vi "PSVCH_Check Double Quotation Marks.vi"(8 "Error In (no error)":errorcluster, 11 "String":string) -> (0 "Error Out":errorcluster, 2 "\"Tag\"[]":string[](array[string]), 3 "Error?":bool)   [LabVIEW 2016]
uses:
  <vilib>/regexp/Match Regular Expression.xnode
panel:
  # "Data In"
  # "Data Out"
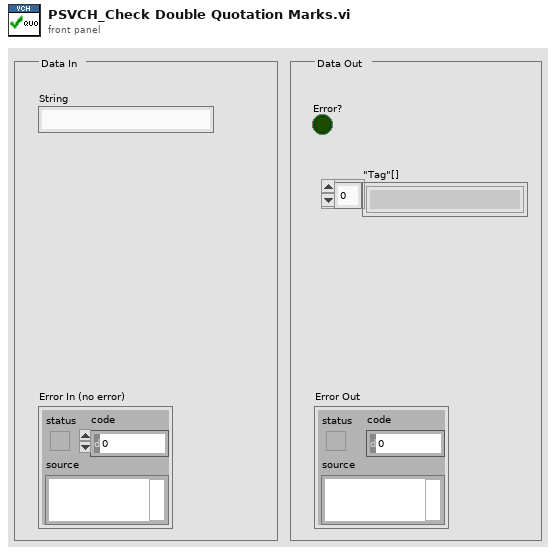
[diagram p1: front panel]
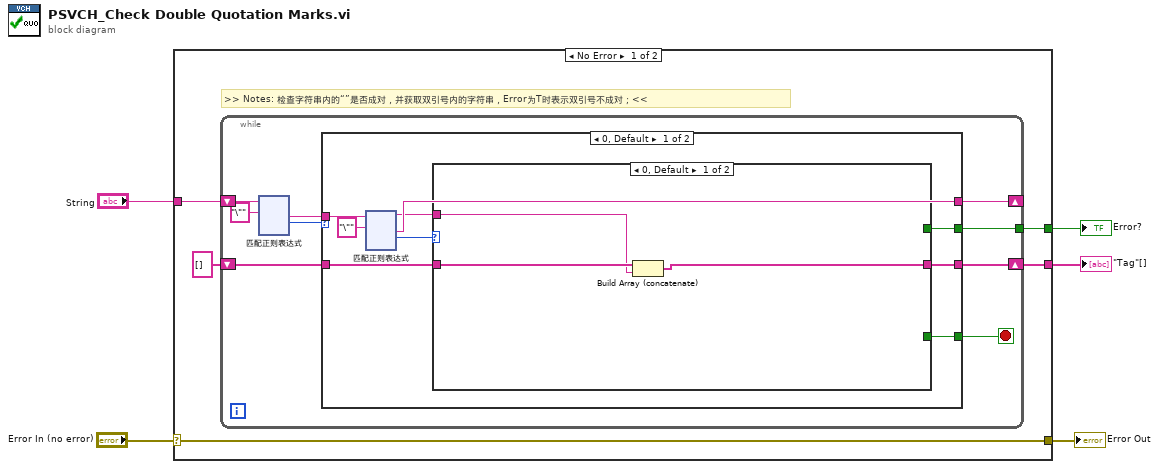
[diagram p0: block diagram]
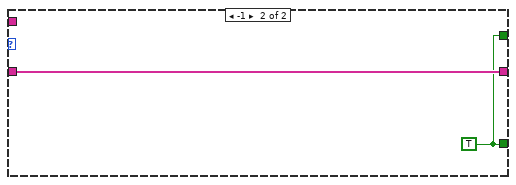
[diagram p2: hidden frame]
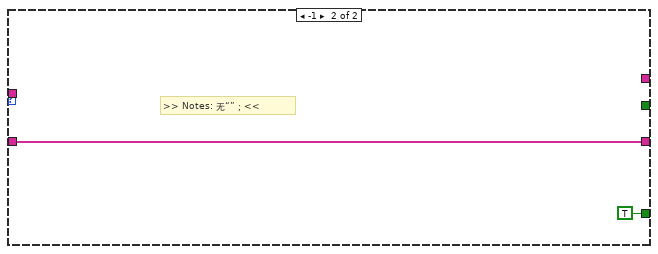
[diagram p3: hidden frame]
diagram:
  n1 = case shown="No Error" "Error In (no error)" {
    selector: "Error In (no error)" -> [w6 w258]
    tunnel: "String" -> [w9 _]
    tunnel: [w8 _] -> w4
    tunnel: [w7 _] -> w3
    tunnel: [w6 w258] -> w1
    frame No Error {
      # ">> Notes: 检查字符串内的“”是否成对，并获取双引号内的字符串，Error为T时表示双引号不成对；<<"
      n2 = while {
        shift-right: [w15] -> _
        shift-left: w9 -> [w19]
        shift-right: [w12] -> w8
        shift-left: string[] [] -> [w13]
        tunnel: [w11] -> w7
        stop <- w14 stop-if-true
        n3 = xnode "匹配正则表达式"("输入字符串"=w19, "正则表达式"="\"") -> ("匹配之后"=w16:string, "匹配后偏移量"=w17:i32)  [unwired: 4 in, 3 out]
        n4 = case shown="0, Default" w17 {
          tunnel: w16 -> [w27 _]
          tunnel: [w25 _] -> w15
          tunnel: [w23 TRUE] -> w14
          tunnel: w13 -> [w22 w146]
          tunnel: [w21 w146] -> w12
          tunnel: [w20 _] -> w11
          frame 0, Default {
            n5 = xnode "匹配正则表达式"("输入字符串"=w27, "正则表达式"="\"") -> ("匹配之前"=w24:string, "匹配之后"=w25:string, "匹配后偏移量"=w26:i32)  [unwired: 4 in, 2 out]
            n6 = case shown="0, Default" w26 {
              tunnel: w24 -> [w30 _]
              tunnel: [_ w32] -> w23
              tunnel: w22 -> [w31 w33]
              tunnel: [w29 w33] -> w21
              tunnel: [_ w32] -> w20
              frame 0, Default {
                n7 = Build Array (concatenate)(w31, w30) -> (w29:string[])
              }
              frame -1 {
                w32 = TRUE
              }
            }
          }
          frame -1 {
            # ">> Notes: 无“”；<<"
          }
        }
      }
    }
    frame Error {
    }
  }
  "\"Tag\"[]" <- w4
  "Error?" <- w3
  "Error Out" <- w1
